vi "Envia serial.vi"(8 "error In":errorcluster, 10 "String a ser Enviado":string, 11 "LNA VISA session (for class)":refnum<visa-resource-name>) -> (0 "error out":errorcluster, 1 "txCount":u32, 2 "String Enviado":string, 3 "LNA VISA session saida":refnum<visa-resource-name>)   [LabVIEW 2018]
uses:
  <vilib>/Instr/_visa.llb/VISA Flush IO Buffer Mask.ctl
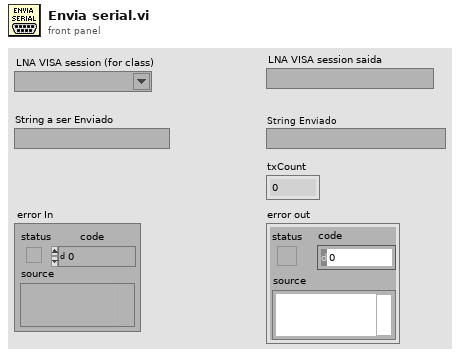
[diagram p1: front panel]
types:
  T1 = typedef "VISA Flush IO Buffer Mask.ctl" = u16
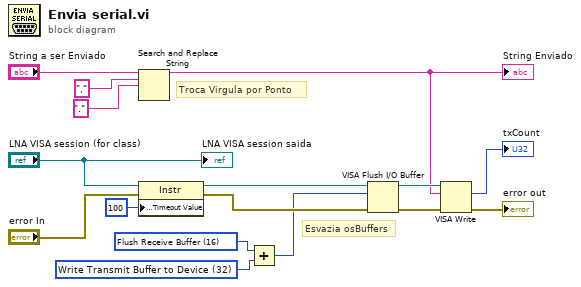
[diagram p0: block diagram]
diagram:
  w9 = T1 32 items=["Flush Receive Buffer"=16, "Write Transmit Buffer to Device"=32, "Flush Receive Buffer (No I/O)"=64, "Flush Transmit Buffer"=128] ("Mask")
  w10 = T1 16 items=["Flush Receive Buffer"=16, "Write Transmit Buffer to Device"=32, "Flush Receive Buffer (No I/O)"=64, "Flush Transmit Buffer"=128] ("Mask")
  # "Esvazia osBuffers"
  # "Troca Virgula por Ponto"
  n1 = Search and Replace String(input string="String a ser Enviado", search string=",", replace string=".") -> (result string=w2:string)  [unwired: 5 in, 3 out]
  "String Enviado" <- w2
  n2 = property class="Instr"(reference="LNA VISA session (for class)", error in="error In", "General Settings:Timeout Value"=u32 100 ("Tmo Value")) -> (reference out=w12:refnum<visa-resource-name>, error out=w11:errorcluster)
  n3 = Add(x=w10, y=w9) -> (x+y=w8:T1)
  n4 = VISA Flush I/O Buffer(VISA resource name=w12, mask (16)=w8, error in (no error)=w11) -> (VISA resource name out=w7:refnum<visa-resource-name>, error out=w6:errorcluster)
  n5 = VISA Write(VISA resource name=w7, write buffer=w2, error in (no error)=w6) -> (return count=→"txCount":u32, error out=→"error out":errorcluster)  [unwired: 1 out]
  "LNA VISA session saida" <- "LNA VISA session (for class)"
